vi "Time_Series.vi"(1 "dt":dbl, 2 "Nsmpls":i32) -> (0 "Times":dbl[](array[numeric]))   [LabVIEW 2019]
doc: "Create an array of time values based on a sample size and a time spacing\nAssumes time t0 = 0\n\nR. Sheehan 11 - 3 - 2020"
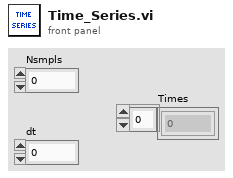
[diagram p1: front panel]
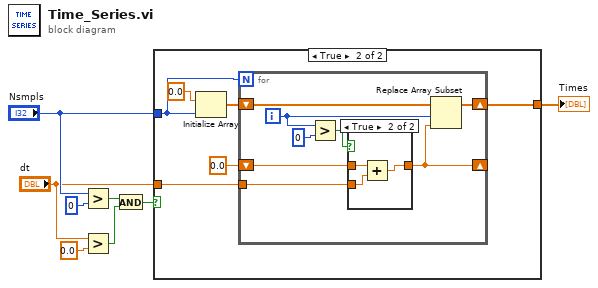
[diagram p0: block diagram]
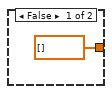
[diagram p2: hidden frame]
diagram:
  n1 = Greater?(x="Nsmpls", y=0) -> (0:w6:bool)
  n2 = Greater?(x="dt", y=0.0) -> (0:w5:bool)
  n3 = And(x=w6, y=w5) -> (x .and. y?=w4:bool)
  n4 = case shown="True" w4 {
    tunnel: "Nsmpls" -> [_ w13]
    tunnel: "dt" -> [_ w15]
    tunnel: [dbl[] [] w11] -> w1
    frame False {
    }
    frame True {
      n5 = Initialize Array(0.0 ("element"), w13) -> (w12:dbl[])
      n6 = for {
        N: w13 -> [_]
        tunnel: w15 -> [w18]
        shift-right: [w22] -> w11
        shift-left: w12 -> [w23]
        shift-right: [w16] -> _
        shift-left: 0.0 -> [w19]
        i -> [w17]
        n7 = Greater?(x=w17, y=0) -> (0:w20:bool)
        n8 = case shown="True" w20 {
          tunnel: [w24 w27] -> w16
          tunnel: w19 -> [w24 w26]
          tunnel: w18 -> [_ w25]
          frame False {
          }
          frame True {
            n9 = Add(x=w26, y=w25) -> (x+y=w27:dbl)
          }
        }
        n10 = Replace Array Subset(array=w23, new element=w16, index=w17) -> (w22:dbl[])
      }
    }
  }
  "Times" <- w1
